vi "Status-Connection-Yaxis.vi"(8 "error in":errorcluster) -> (0 "error out":errorcluster)   [LabVIEW 2014, in "Motion-ControlAll.lvclass"]
uses:
  Motion-ControlAll.lvclass
  <vilib>/Utility/error.llb/Error Cluster From Error Code.vi
  <vilib>/ErrorRing/Error Ring.xnode
panel:
  in  "Continue":bool
  in  "String":string="The Y-Axis Motor Controller Did not Establish Communication. \n\nPlease Press the QUIT Button and troubleshoot the problem. \n\n1. Unplug the Power to the Y-Axis Motor Controller from the power strip located on the floor. \n\n2. Unplug the USB hub located on the front of the computer. Unplug and Plug back into the EXACT PORT it was unplugged from. "
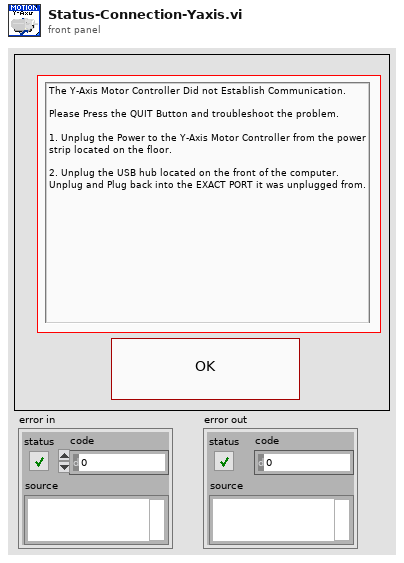
[diagram p1: front panel]
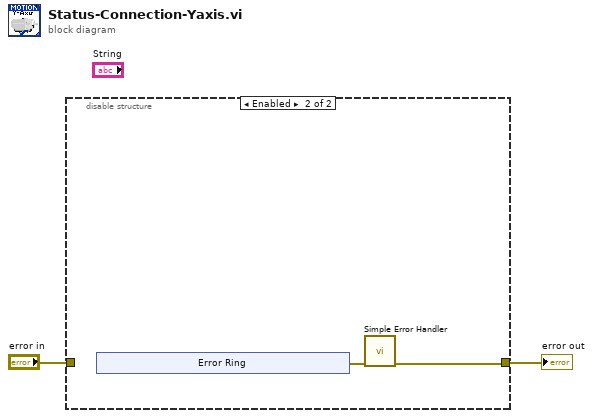
[diagram p0: block diagram]
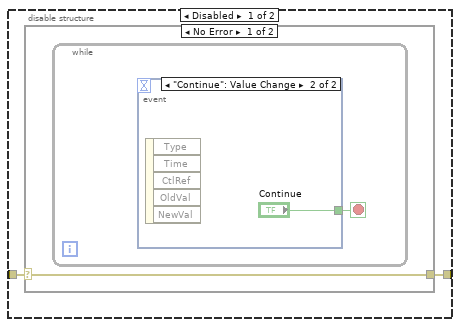
[diagram p2: hidden frame]
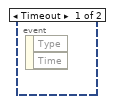
[diagram p3: hidden frame]
diagram:
  n1 = disable-structure shown="Enabled" {
    disable-tunnel: "error in" -> [w4 _]
    disable-tunnel: [w3 w9] -> w1
    frame Disabled {
      n2 = case shown="No Error" w4 {
        selector: w4 -> [w5 w8]
        tunnel: [w5 w8] -> w3
        frame No Error {
          n3 = while {
            stop <- w6 stop-if-true
            n4 = event shown="[1] \"Continue\": Value Change" {
              selector: _ -> [_ _]
              dyn-events: _ -> [_ _]
              timeout: _ -> [_ _]
              tunnel: [_ "Continue"] -> w6
              event Timeout {
                n5 = event-data() -> ()  [unwired: 1 in, 2 out]
              }
              event "Continue": Value Change {
                n6 = event-data() -> ()  [unwired: 1 in, 5 out]
              }
            }
          }
        }
        frame Error {
        }
      }
    }
    frame Enabled {
      n7 = xnode "Error Ring"() -> ("error out"=w10:errorcluster)
      n8 = call <vilib>:"Simple Error Handler.vi"("error in (no error)"=w10) -> ("error out"=w9:errorcluster)  [unwired: 4 in, 4 out]
    }
  }
  "error out" <- w1
